vi "Get Thermocouple Detection.vi"(8 "error in (no error)":errorcluster, 11 "VISA resource name":refnum<visa-resource-name>) -> (0 "error out":errorcluster, 2 "Thermocouple Detection":u16, 3 "VISA resource name out":refnum<visa-resource-name>)   [LabVIEW 2011, in "Fluke 5XXX Series Multicalibrators.lvlib"]
doc: "This VI returns the status of the open thermocouple detection circuit in thermocouple measurement mode.\n\nNote:\n\nThis VI is available only for instrument models 5500A and 5520A."
uses:
  Fluke 5XXX Series Multicalibrators.lvlib
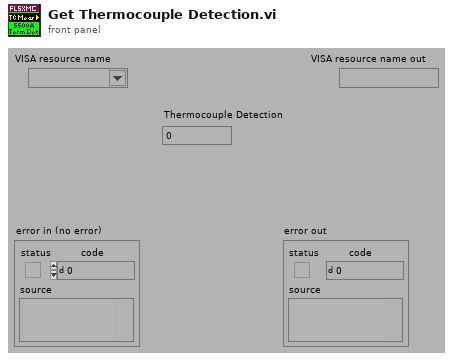
[diagram p1: front panel]
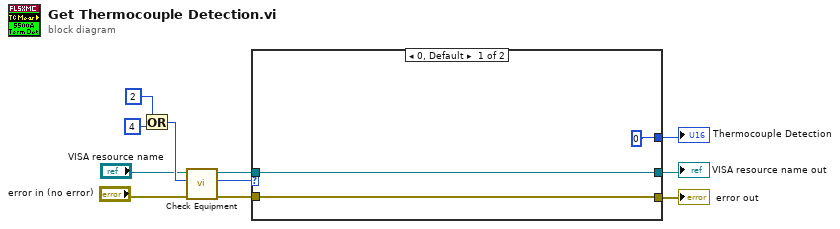
[diagram p0: block diagram]
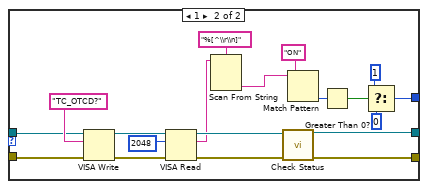
[diagram p2: hidden frame]
diagram:
  n1 = Or(x=2 ("Numeric"), y=4 ("Numeric")) -> (x .or. y?=w7:i32)
  n2 = call "Check Equipment.vi"("error in (no error)"="error in (no error)", "Bit Mask"=w7, "VISA resource name"="VISA resource name") -> ("error out"=w11:errorcluster, "Present?"=w9:u32, "VISA resource name out"=w10:refnum<visa-resource-name>)  [unwired: 6 in]
  n3 = case shown="0, Default" w9 {
    tunnel: [w14 w27] -> w4
    tunnel: [w13 w24] -> w3
    tunnel: w11 -> [w14 w29]
    tunnel: w10 -> [w13 w28]
    tunnel: [u16 0 w16] -> w2
    frame 0, Default {
    }
    frame 1 {
      n4 = VISA Write(VISA resource name=w28, write buffer="TC_OTCD?", error in (no error)=w29) -> (VISA resource name out=w32:refnum<visa-resource-name>, error out=w31:errorcluster)  [unwired: 1 out]
      n5 = VISA Read(VISA resource name=w32, byte count=u32 2048 ("byte count (0)"), error in (no error)=w31) -> (VISA resource name out=w25:refnum<visa-resource-name>, read buffer=w22:string, error out=w26:errorcluster)  [unwired: 1 out]
      n6 = Scan From String(format string="%[^\\r\\n]", input string=w22) -> (output 1=w15:string)  [unwired: 3 in, 3 out]
      n7 = call "Check Status.vi"("VISA resource name"=w25, "error in (no error)"=w26) -> ("VISA resource name out"=w24:refnum<visa-resource-name>, "error out"=w27:errorcluster)  [unwired: 12 in]
      n8 = Match Pattern(string=w15, regular expression="ON") -> (offset past match=w20:i32)  [unwired: 1 in, 3 out]
      n9 = Greater Than 0?(x=w20) -> (x > 0?=w17:bool)
      n10 = Select(t=u16 1 ("f"), s=w17, f=u16 0) -> (s? t:f=w16:u16)
    }
  }
  "Thermocouple Detection" <- w2
  "VISA resource name out" <- w3
  "error out" <- w4
